vi "rmViFromLib.vi"(8 "error in (no error)":errorcluster, 10 "arrayOfVi":path[](array[path]), 11 "libRefIn":refnum<vi>) -> (0 "error out":errorcluster, 3 "libRefInOut":refnum<vi>)   [LabVIEW 2018]
doc: "Remove the vi files from LabVIEW library."
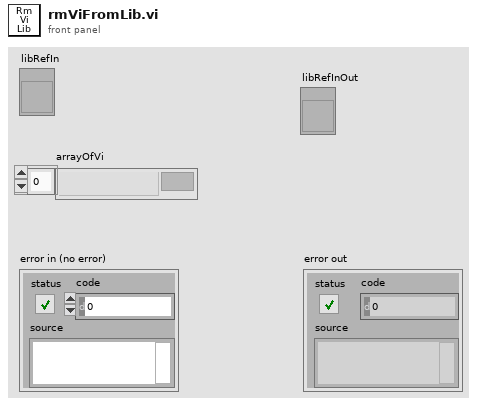
[diagram p1: front panel]
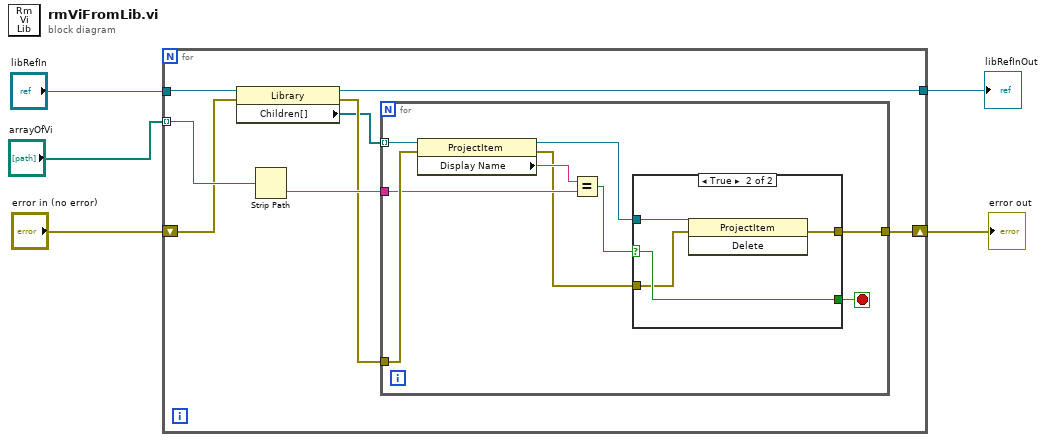
[diagram p0: block diagram]
diagram:
  n1 = for {
    shift-right: [w10] -> w4
    shift-left: "error in (no error)" -> [w9]
    tunnel: "libRefIn" -> [w13]
    tunnel: "arrayOfVi" -> [w12] mode=indexing
    tunnel: [w6] -> w1
    n2 = property class="Library"(reference=w13, error in=w9) -> (reference out=w6:refnum<vi>, error out=w8:errorcluster, "Children[]"=w7:refnum<vi>[])
    n3 = Strip Path(path=w12) -> (name=w11:string)  [unwired: 1 out]
    n4 = for {
      tunnel: w7 -> [w22] mode=indexing
      tunnel: w8 -> [w21]
      tunnel: w11 -> [w19]
      tunnel: [w14] -> w10
      stop <- w17 stop-if-true
      n5 = property class="ProjectItem"(reference=w22, error in=w21) -> (reference out=w16:refnum<vi>, error out=w15:errorcluster, "Display Name"=w20:string)
      n6 = Equal?(x=w20, y=w19) -> (x = y?=w18:bool)
      n7 = case shown="True" w18 {
        selector: w18 -> [w24 w28]
        tunnel: [w24 w28] -> w17
        tunnel: w16 -> [_ w27]
        tunnel: w15 -> [w23 w26]
        tunnel: [w23 w25] -> w14
        frame False {
        }
        frame True {
          n8 = invoke class="ProjectItem" method="Delete"(reference=w27, error in=w26) -> (error out=w25:errorcluster)  [unwired: 1 in, 2 out]
        }
      }
    }
  }
  "error out" <- w4
  "libRefInOut" <- w1
